vi "Get Elapsed Times.vi"(8 "error in":errorcluster, 11 "Path":path) -> (0 "error out":errorcluster, 3 "Elapsed Times":dbl[](array[numeric]))   [LabVIEW 2019]
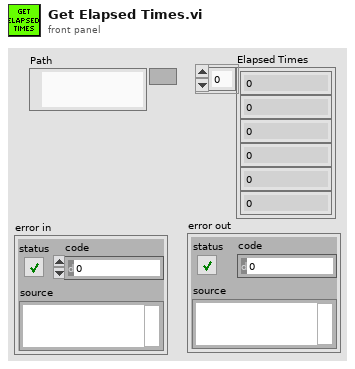
[diagram p1: front panel]
types:
  T1 = enum16{"open", "replace", "create", "open or create", "replace or create", "replace or create with confirmation"}
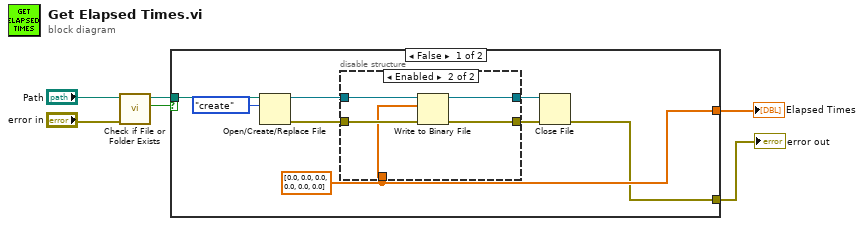
[diagram p0: block diagram]
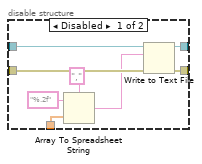
[diagram p2: hidden frame]
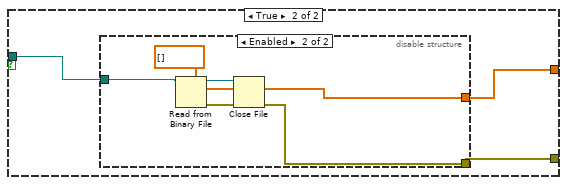
[diagram p3: hidden frame]
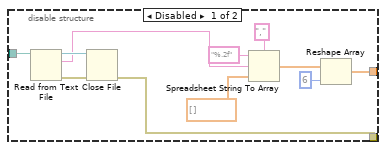
[diagram p4: hidden frame]
diagram:
  n1 = call <vilib>:"Check if File or Folder Exists.vi"("error in (no error)"="error in", "path"="Path") -> ("file or folder exists?"=w1:bool, "dup path"=w4:path)  [unwired: 7 in, 1 out]
  n2 = case shown="False" w1 {
    tunnel: w4 -> [w14 w30]
    tunnel: [w13 w29] -> w3
    tunnel: [w10 w28] -> w2
    frame False {
      w13 = dbl[] [0.0, 0.0, 0.0, 0.0, 0.0, 0.0]
      n3 = Open/Create/Replace File(file path (use dialog)=w14, operation (0:open)=T1."create") -> (refnum out=w8:refnum<file>, error out=w7:errorcluster)  [unwired: 4 in, 1 out]
      n4 = disable-structure shown="Enabled" {
        disable-tunnel: w13 -> [w20 w23]
        disable-tunnel: [w19 w24] -> w12
        disable-tunnel: [w18 w26] -> w11
        disable-tunnel: w8 -> [w17 w27]
        disable-tunnel: w7 -> [w16 w25]
        frame Disabled {
          n5 = Array To Spreadsheet String(delimiter (Tab)=",", array=w20, 3:"%.2f" ("format string")) -> (spreadsheet string=w15:string)
          n6 = Write to Text File(file (use dialog)=w17, text=w15, error in=w16) -> (refnum out=w18:refnum<file>, error out=w19:errorcluster)  [unwired: 1 in, 1 out]
        }
        frame Enabled {
          n7 = Write to Binary File(file (use dialog)=w27, data=w23, error in=w25) -> (refnum out=w26:refnum<file>, error out=w24:errorcluster)  [unwired: 3 in, 1 out]
        }
      }
      n8 = Close File(refnum=w11, error in=w12) -> (error out=w10:errorcluster)  [unwired: 1 out]
    }
    frame True {
      n9 = disable-structure shown="Enabled" {
        disable-tunnel: w30 -> [w33 w47]
        disable-tunnel: [w32 w45] -> w29
        disable-tunnel: [w31 w42] -> w28
        frame Disabled {
          n10 = Read from Text File(file (use dialog)=w33) -> (refnum out=w35:refnum<file>, text=w34:string, error out=w36:errorcluster)  [unwired: 3 in, 1 out]
          n11 = Close File(refnum=w35, error in=w36) -> (error out=w31:errorcluster)  [unwired: 1 out]
          n12 = Spreadsheet String To Array(delimiter (Tab)=",", format string="%.2f", spreadsheet string=w34, array type (2D Dbl)=dbl[] []) -> (array=w40:dbl[])
          n13 = Reshape Array(w40, 6 ("dimension size")) -> (w32:dbl[])
        }
        frame Enabled {
          n14 = Read from Binary File(5:dbl[] [], 11:w47) -> (0:w43:errorcluster, 2:w45:dbl[], 3:w44:refnum<file>)  [unwired: 4 in, 1 out]
          n15 = Close File(refnum=w44, error in=w43) -> (error out=w42:errorcluster)  [unwired: 1 out]
        }
      }
    }
  }
  "Elapsed Times" <- w3
  "error out" <- w2
